vi "Analysis.Main.vi"(8 "error in (no error)":errorcluster, 9 "Refs":T2, 10 "Data Path":path, 11 "Parameters":T1={"Results Path"=path "C:/Conti/Logs", "Temp Path"=path "C:/Conti/Temp", "Remote Path"=path "d:/Conti/Logs", "Analysis VIs"=[], "Report Passed?"=FALSE, "Group Channels?"=FALSE}) -> (0 "error out":errorcluster, 3 "Overall Result":bool)   [LabVIEW 2015, in "NIAnalysis.lvlib"]
uses:
  NIAnalysis.lvlib
  Types/AnalysisGUI.Refs.ctl
  Types/AnalysisGUI.Parameters.ctl
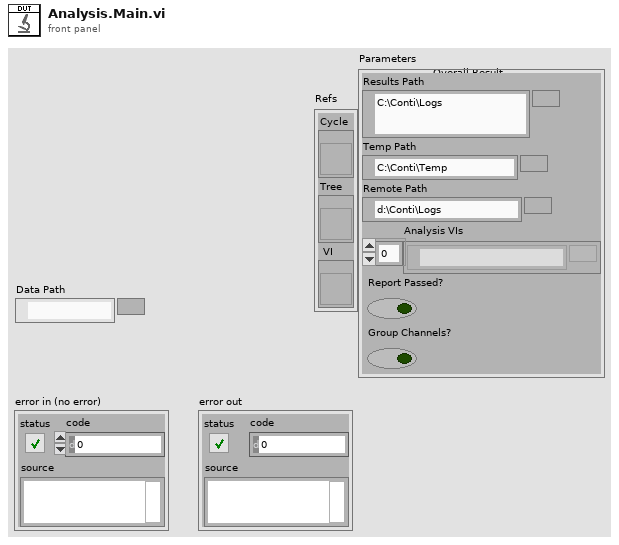
[diagram p1: front panel]
types:
  T1 = typedef "NIAnalysis.lvlib/AnalysisGUI.Parameters.ctl" = cluster{"Results Path":path, "Temp Path":path, "Remote Path":path, "Analysis VIs":path[], "Report Passed?":bool, "Group Channels?":bool}
  T2 = typedef "NIAnalysis.lvlib/AnalysisGUI.Refs.ctl" = cluster{"Cycle":refnum<vi>, "Tree":refnum<vi>, " VI":refnum<vi>}
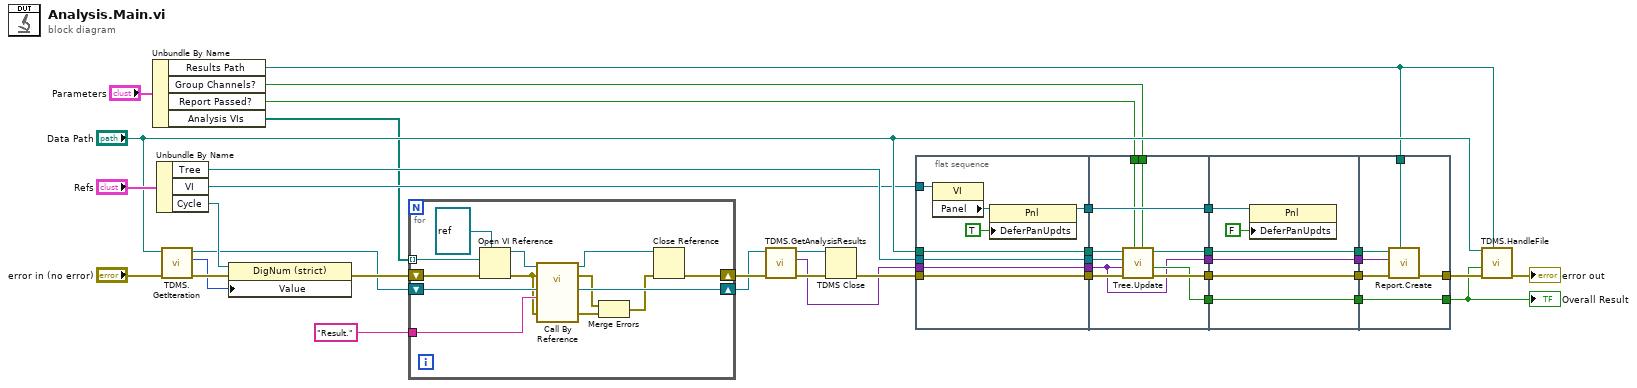
[diagram p0: block diagram]
diagram:
  n1 = Unbundle By Name("Parameters") -> ("Results Path"=w3:path, "Group Channels?"=w2:bool, "Report Passed?"=w10:bool, "Analysis VIs"=w11:path[])
  n2 = Unbundle By Name("Refs") -> ("Tree"=w27:refnum<vi>, "VI"=w19:refnum<vi>, "Cycle"=w37:refnum<vi>)
  n3 = call "TDMS.GetIteration.vi"("error in (no error)"="error in (no error)", "Data"="Data Path") -> ("error out"=w36:errorcluster, "Iteration"=w35:i32, "tdms file out"=w14:refnum<k34>)  [unwired: 7 in]
  n4 = property class="DigNum (strict)"(reference=w37, error in=w36, "Value"=w35) -> (error out=w16:errorcluster)  [unwired: 1 out]
  n5 = for {
    tunnel: "Result." ("Result.Prefix") -> [w50]
    shift-right: [w47] -> w15
    shift-left: w16 -> [w49]
    shift-right: [w45] -> w13
    shift-left: w14 -> [w46]
    tunnel: w11 -> [w40] mode=indexing
    n6 = Open VI Reference(type specifier VI Refnum (for type only)=refnum<vi> refnum, vi path=w40, error in (no error)=w49) -> (vi reference=w52:refnum<vi>, error out=w44:errorcluster)  [unwired: 3 in]
    n7 = call-by-ref "?"(reference=w52, error in=w44, "error in"=w44, "Result.Prefix"=w50, "tdms file"=w46) -> (reference out=w48:refnum<vi>, error out=w42:errorcluster, 0:"error out"=w43:errorcluster, "tdms file out"=w45:refnum<k34>)  [unwired: 7 in]
    n8 = Merge Errors(w42, w43) -> (w41:errorcluster)
    n9 = Close Reference(reference=w48, error in (no error)=w41) -> (error out=w47:errorcluster)
  }
  n10 = call "TDMS.GetAnalysisResults.vi"("error in (no error)"=w15, "Refnum in"=w13) -> ("error out"=w32:errorcluster, "Variant"=w28:variant, "Refnum out"=w31:refnum<k34>)  [unwired: 7 in]
  n11 = TDMS Close(8:w32, 11:w31) -> (0:w30:errorcluster)  [unwired: 1 out]
  n12 = flat-sequence {
    tunnel: "Data Path" -> [w57]
    tunnel: w27 -> [w58]
    tunnel: w28 -> [w59]
    tunnel: w30 -> [w60]
    tunnel: [w60] -> w25
    tunnel: [w59] -> w24
    tunnel: [w58] -> w23
    tunnel: [w57] -> w22
    tunnel: w19 -> [w54]
    tunnel: [w53] -> w17
    tunnel: w25 -> [w69]
    tunnel: w24 -> [w62]
    tunnel: w23 -> [w67]
    tunnel: w22 -> [w66]
    tunnel: [w70] -> w21
    tunnel: [w68] -> w20
    tunnel: [w65] -> w18
    tunnel: w17 -> [w65]
    tunnel: w10 -> [w64]
    tunnel: [w63] -> w6
    tunnel: [w62] -> w5
    tunnel: w2 -> [w61]
    tunnel: w21 -> [w76]
    tunnel: w20 -> [w75]
    tunnel: w18 -> [w74]
    tunnel: [w76] -> w9
    tunnel: [w75] -> w8
    tunnel: [w72] -> w7
    tunnel: w6 -> [w72]
    tunnel: w5 -> [w71]
    tunnel: [w71] -> w4
    tunnel: [w82] -> w29
    tunnel: [w80] -> w34
    tunnel: w9 -> [w81]
    tunnel: w8 -> [w82]
    tunnel: w7 -> [w79]
    tunnel: w4 -> [w78]
    tunnel: w3 -> [w77]
    frame #0 {
      n13 = property class="VI"(reference=w54) -> ("Panel"=w55:refnum<vi>)  [unwired: 1 in, 2 out]
      n14 = property class="Pnl"(reference=w55, "DeferPanUpdts"=TRUE ("Defer Panel Updates")) -> (reference out=w53:refnum<vi>)  [unwired: 1 in, 1 out]
    }
    frame #1 {
      n15 = call "Tree.Update.vi"("Group Channels?"=w61, "Report Passed?"=w64, "error in (no error)"=w69, "Results"=w62, "TreeControl in"=w67, "Data Path"=w66) -> ("error out"=w70:errorcluster, "Passed?"=w68:bool, "Data Path"=w63:path)  [unwired: 2 in, 1 out]
    }
    frame #2 {
      n16 = property class="Pnl"(reference=w74, "DeferPanUpdts"=FALSE ("Defer Panel Updates")) -> ()  [unwired: 1 in, 2 out]
    }
    frame #3 {
      n17 = call "Report.Create.vi"("Result Directory"=w77, "error in (no error)"=w81, "Results"=w78, "Data Path"=w79) -> ("error out"=w80:errorcluster)  [unwired: 7 in]
    }
  }
  n18 = call "TDMS.HandleFile.vi"("Result Directory"=w3, "error out"=w34, "Delete"=w29, "Data"="Data Path") -> ("error out"=→"error out":errorcluster)  [unwired: 6 in, 1 out]
  "Overall Result" <- w29
